vi "Create.vi"(6 "Upper Red Threshold":dbl, 8 "Upper Green Threshold":dbl, 9 "Lower Green Threshold":dbl, 10 "Lower Red Threshold":dbl) -> (3 "Aim Middle Threshold out":refnum<class "Aim Middle Threshold.lvclass">)   [LabVIEW 2021, in "Aim Middle Threshold.lvclass"]
uses:
  Aim Middle Threshold.lvclass
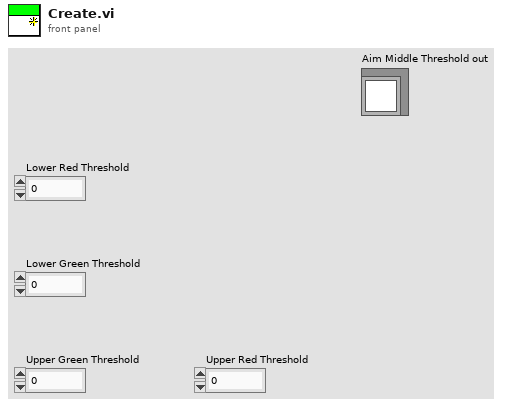
[diagram p1: front panel]
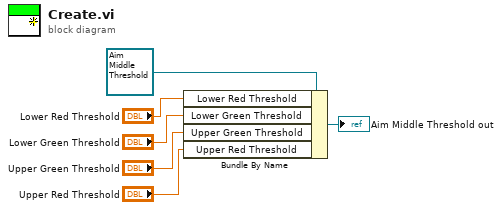
[diagram p0: block diagram]
diagram:
  n1 = Bundle By Name(cluster=refnum<class "Aim Middle Threshold.lvclass"> refnum ("Aim Middle Threshold in"), "Lower Red Threshold"="Lower Red Threshold", "Lower Green Threshold"="Lower Green Threshold", "Upper Green Threshold"="Upper Green Threshold", "Upper Red Threshold"="Upper Red Threshold") -> (→"Aim Middle Threshold out":refnum<class "Aim Middle Threshold.lvclass">)
